vi "pause_after_iteration.vi"(8 "error in (no error)":errorcluster) -> (0 "error out":errorcluster)   [LabVIEW 2013]
uses:
  <vilib>/Platform/TimedLoop/XDataNode/wakeup.ctl
  <vilib>/Platform/TimedLoop/XDataNode/XDNodeRunTimeDep.lvlib
  <vilib>/Platform/TimedLoop/XDataNode/nitl_modes.ctl
  <vilib>/Platform/TimedLoop/XDataNode/timing_clust.ctl
  <vilib>/platform/TimedLoop/XDataNode/XDataNode.xnode
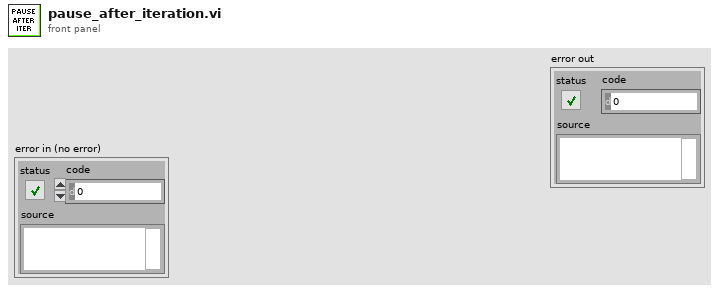
[diagram p1: front panel]
types:
  T1 = typedef "XDNodeRunTimeDep.lvlib/timing_clust.ctl" = cluster{"Expected End [f-1]":u64, "Actual End [f-1]":u64, "Finished Late? [f-1]":bool, "Expected End [i-1]":u64, "Actual End [i-1]":u64, "Finished Late? [i-1]":bool, "Expected Start [i]":u64, "Actual Start [i]":u64, "Expected Start [f]":u64, "Actual Start [f]":u64, "Source Name":string, "Structure Name":string, "Period":i64, "Deadline":i64, "Offset":i64, "Start":i64, "Priority":i32, "Timeout":i32, "Mode":T2, "Wakeup Reason":T3, "Error":errorcluster, "Source Type":string, "Secondary Source Type":string, "Global End Time":u64, "Global Start Time":u64, "Frame Duration":u64, "Iteration Duration":u64, "Assigned CPU":i32, "I/O Scan Engine Mode":u32}
  T2 = typedef "XDNodeRunTimeDep.lvlib/nitl_modes.ctl" = enum32{"No Change", "Process missed periods, maintain original phase", "Discard missed periods, maintain original phase", "Process missed periods, ignore original phase", "Discard missed periods, ignore original phase"}
  T3 = typedef "XDNodeRunTimeDep.lvlib/wakeup.ctl" = enum32{"Normal", "Aborted", "Asynchronous wakeup", "Timing source error", "Timed loop error", "Timeout"}
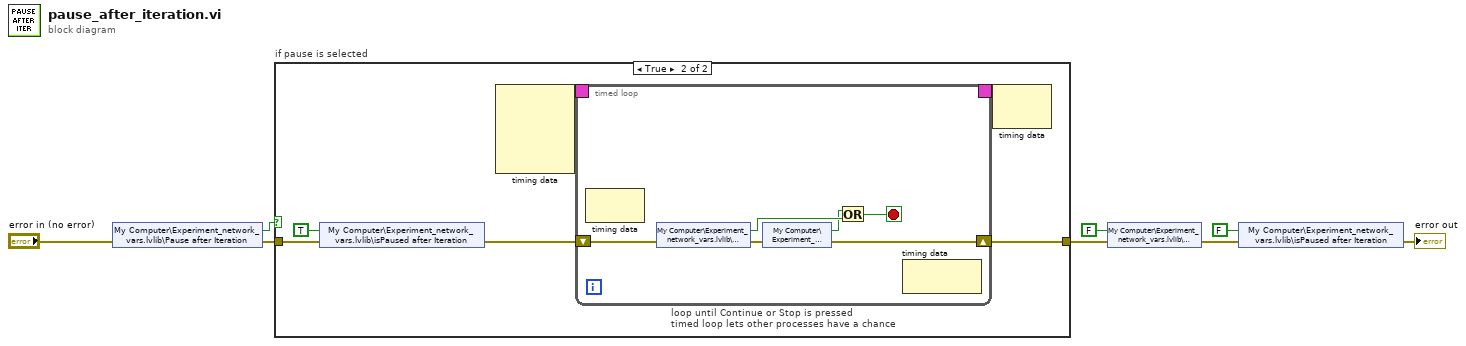
[diagram p0: block diagram]
diagram:
  n1 = shared-variable "My Computer\\Experiment_network_vars.lvlib\\Pause after Iteration"(error in="error in (no error)") -> (w8:bool, error out=w7:errorcluster)
  n2 = case "if pause is selected" shown="True" w8 {
    tunnel: w7 -> [w9 w14]
    tunnel: [w9 w12] -> w2
    frame False {
    }
    frame True {
      n3 = shared-variable "My Computer\\Experiment_network_vars.lvlib\\isPaused after Iteration"(TRUE ("isPaused after Measurement"), error in=w14) -> (error out=w13:errorcluster)
      n4 = node-c288() -> (w11:T1)  [unwired: 4 in]
      n5 = timed-loop "loop until Continue or Stop is pressed\ntimed loop lets other processes have a chance" {
        shift-right: [w16] -> w12
        shift-left: w13 -> [w21]
        timing: w11 -> [_]
        timing-out: [_] -> w10
        stop <- w18 stop-if-true
        n6 = node-c288() -> ()  [unwired: 1 in, 1 out]
        n7 = shared-variable "My Computer\\Experiment_network_vars.lvlib\\Continue"(error in=w21) -> (w20:bool, error out=w17:errorcluster)
        n8 = shared-variable "My Computer\\Experiment_network_vars.lvlib\\Stop"(error in=w17) -> (w19:bool, error out=w16:errorcluster)
        n9 = Or(x=w19, y=w20) -> (x .or. y?=w18:bool)
        n10 = node-c288() -> ()  [unwired: 1 in, 1 out]
      }
      n11 = node-c288(w10) -> ()  [unwired: 1 out]
    }
  }
  n12 = shared-variable "My Computer\\Experiment_network_vars.lvlib\\Continue"(FALSE ("Continue"), error in=w2) -> (error out=w1:errorcluster)
  n13 = shared-variable "My Computer\\Experiment_network_vars.lvlib\\isPaused after Iteration"(FALSE ("isPaused after Measurement"), error in=w1) -> (error out=→"error out":errorcluster)
